vi "Data_to_uart_format.vi"(2 "Payload  Byte to be sent":u8[](array[numeric]), 3 "Types of Data":T1, 4 "MCU Address to be sent":T2) -> (0 "Byte array has been sent":u8[](array[numeric]), 1 "Converted Message":string)   [LabVIEW 2016]
doc: "The funksjon of this VI is to format you data to a string for the Embedded smart home format.\nThere are 3 inputs and 1 important output. There is also an addition input for view what has been sent.\n\nInput 1: MCU Adress\nInput 2: Message Type\nInput 3: Payload\nOuput 1: String to be sent to UART\n(option) Output 2: Array of the bytes being sent"
uses:
  Typedef/MCU_addresses.ctl
  Typedef/Type_of_message_to_MCU.ctl
panel:
  out "Types of Data 2":T1
  out "Size of payload":i32
  out "Payload":u8[](array[numeric])
  in  "Intial array":u8[](array[numeric])
  out "MCU address":string
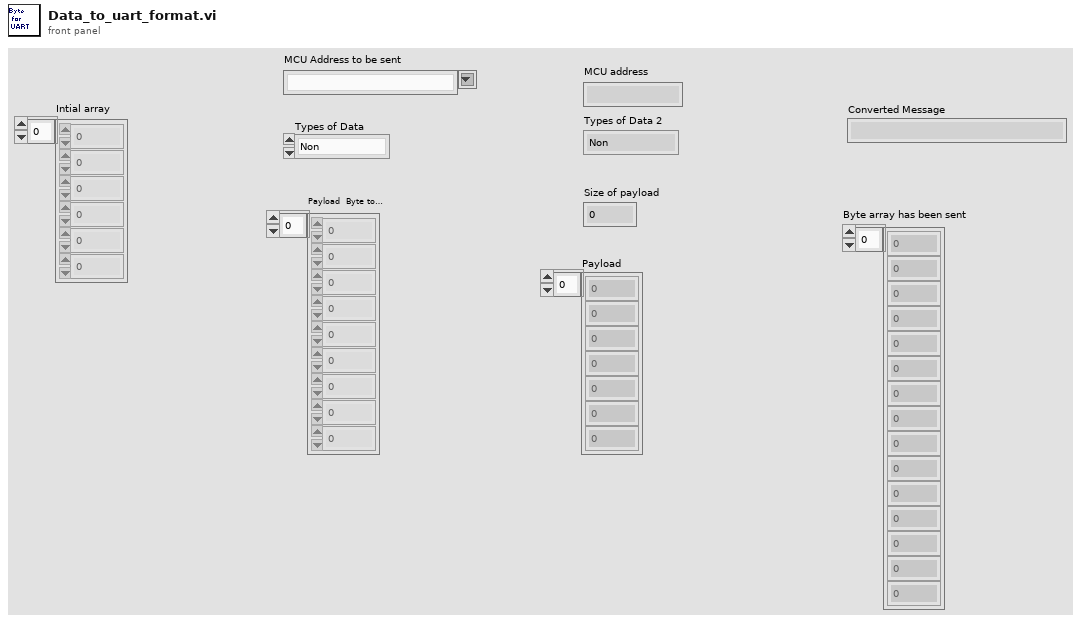
[diagram p1: front panel]
types:
  T1 = typedef "Type_of_message_to_MCU.ctl" = enum16{"Non", "Alarm", "Error", "Time and Date", "Status", "Request"}
  T2 = typedef "MCU_addresses.ctl" = string
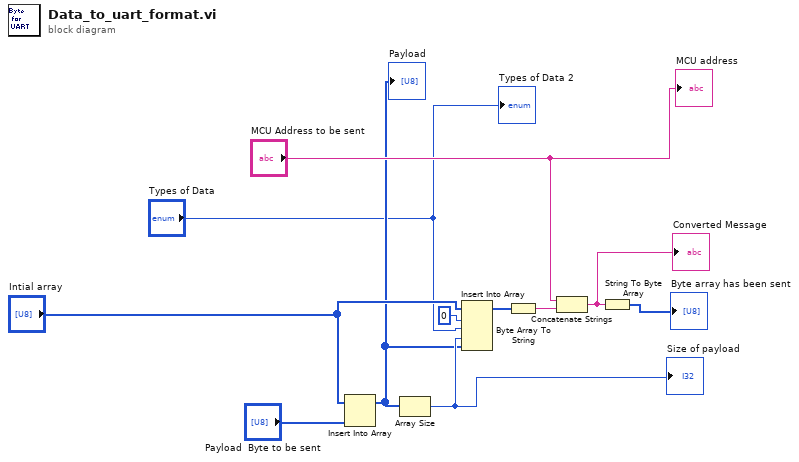
[diagram p0: block diagram]
diagram:
  n1 = Insert Into Array(array="Intial array", new element="Payload  Byte to be sent") -> (w2:u8[])  [unwired: 1 in]
  "Payload" <- w2
  n2 = Array Size(array=w2) -> (size(s)=w7:i32)
  "Size of payload" <- w7
  n3 = Insert Into Array(array="Intial array", index=u8 0, new element #1="Types of Data", new element #2=w7, new element #3=w2) -> (w8:u8[])
  n4 = Byte Array To String(unsigned byte array=w8) -> (string=w9:string)
  n5 = Concatenate Strings("MCU Address to be sent", w9) -> (w5:string)
  "Converted Message" <- w5
  n6 = String To Byte Array(string=w5) -> (unsigned byte array=→"Byte array has been sent":u8[])
  "MCU address" <- "MCU Address to be sent"
  "Types of Data 2" <- "Types of Data"
